vi "SetSoundVeloc.vi"(8 "错误输入（无错误）":errorcluster, 10 "材料声速":u32) -> (0 "错误输出":errorcluster)   [LabVIEW 2014]
uses:
  X86Dll/ZXUTConfigMgr.dll
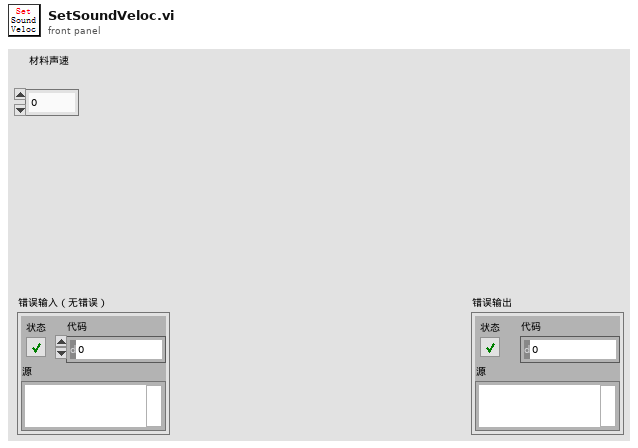
[diagram p1: front panel]
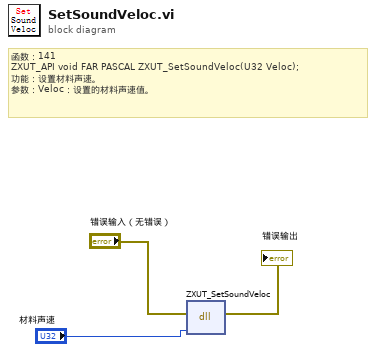
[diagram p0: block diagram]
diagram:
  # "函数：141\nZXUT_API void\tFAR PASCAL ZXUT_SetSoundVeloc(U32 Veloc);\n功能：设置材料声速。\n参数：Veloc：设置的材料声速值。"
  n1 = dll-call lib="D:/Software/Utrasonic on-line monitoring/X86Dll/ZXUTConfigMgr.dll" fn="ZXUT_SetSoundVeloc"(error in="错误输入（无错误）", "Veloc"="材料声速") -> (error out=→"错误输出":errorcluster)  [unwired: 4 in, 1 out]
